vi "tituloDoArquivo.vi"(6 "area":i16 caption="Área da célula", 8 "temperatura":i16 caption="Temperatura da célula", 9 "Tipo":string caption="Tipo da célula", 10 "Nome da célula":string, 11 "file path (dialog if empty)":path) -> ()   [LabVIEW 2012]
uses:
  <vilib>/Utility/file.llb/Write To Spreadsheet File (string).vi
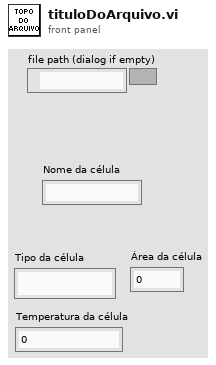
[diagram p1: front panel]
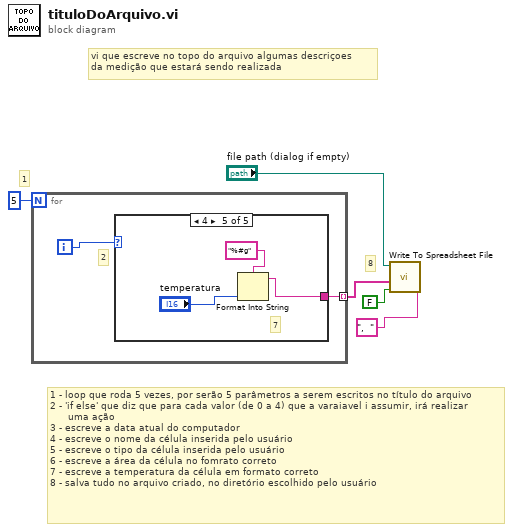
[diagram p0: block diagram]
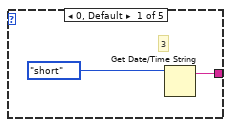
[diagram p2: hidden frame]
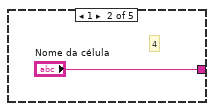
[diagram p3: hidden frame]
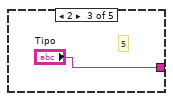
[diagram p4: hidden frame]
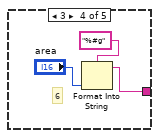
[diagram p5: hidden frame]
diagram:
  # "vi que escreve no topo do arquivo algumas descriçoes\nda medição que estará sendo realizada"
  # "1 - loop que roda 5 vezes, por serão 5 parâmetros a serem escritos no título do arquivo\n2 - 'if else' que diz que para cada valor (de 0 a 4) que a varaiavel i assumir, irá realizar\n      uma ação \n3 - escreve a data atual do computador\n4 - escreve o nome da célula inserida pelo usuário \n5 - escreve o tipo da célula inserida pelo usuário \n6 - escreve a área da célula no fomrato correto \n7 - escreve a temperatura da célula em formato correto \n8 - salva tudo no arquivo criado, no diretório escolhido pelo usuário"
  # "8"
  # "1"
  n1 = for {
    N: 5 -> [_]
    tunnel: [w7] -> w5 mode=indexing
    i -> [w6]
    # "2"
    n2 = case shown="4" w6 {
      tunnel: [w9 "Nome da célula" "Tipo" w13 w16] -> w7
      frame 0, Default {
        # "3"
        n3 = Get Date/Time String(date format (0)=enum16{"short", "long", "abbreviated"}."short") -> (date string=w9:string)  [unwired: 2 in, 1 out]
      }
      frame 1 {
        # "4"
      }
      frame 2 {
        # "5"
      }
      frame 3 {
        # "6"
        n4 = Format Into String(format string="%#g", "area") -> (resulting string=w13:string)  [unwired: 2 in, 1 out]
      }
      frame 4 {
        # "7"
        n5 = Format Into String(format string="%#g", "temperatura") -> (resulting string=w16:string)  [unwired: 2 in, 1 out]
      }
    }
  }
  n6 = call-poly <vilib>:"Write To Spreadsheet File.vi"("delimiter (\\t)"=",  " ("delimiter (\\t)"), "append to file? (new file:F)"=FALSE, "1D data"=w5, "file path (dialog if empty)"="file path (dialog if empty)") -> ()  [unwired: 4 in, 1 out]
